vi "String to Bool.vi"(8 "error in":errorcluster, 11 "Integer String":string) -> (0 "error out":errorcluster, 3 "Bool":bool)   [LabVIEW 2024, in "Electronic Datasheet.lvlib"]
doc: "A string that contains the number to convert."
uses:
  Core/Electronic Datasheet.lvlib
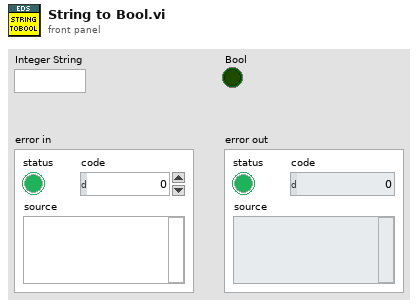
[diagram p1: front panel]
types:
  T1 = enum16{"U8", "U16", "U32", "I8", "I16", "I32", "Bool"}
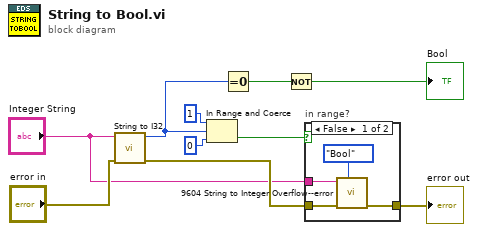
[diagram p0: block diagram]
diagram:
  n1 = call "String to I32.vi"("error in"="error in", "Integer String"="Integer String") -> ("error out"=w7:errorcluster, "I32"=w5:i32)  [unwired: 8 in]
  n2 = In Range and Coerce(upper limit=1, x=w5, lower limit=0) -> (In Range?=w8:bool)  [unwired: 1 out]
  n3 = Equal To 0?(x=w5) -> (x = 0?=w4:bool)
  n4 = Not(x=w4) -> (.not. x?=→"Bool":bool)
  n5 = case "in range?" shown="False" w8 {
    tunnel: w7 -> [w14 w15]
    tunnel: [w13 w15] -> w6
    tunnel: "Integer String" -> [w12 _]
    frame False {
      n6 = call "9604 String to Integer Overflow--error.vi"("Type"=T1."Bool", "error in"=w14, "Integer String"=w12) -> ("error out"=w13:errorcluster)  [unwired: 8 in]
    }
    frame True {
    }
  }
  "error out" <- w6
